vi "GT Get Kvff Filter.vi"(6 "pAccMax":dbl, 7 "pKvffFilterExp":i16, 8 "error in (no error)":errorcluster caption="错误输入（无错误）", 9 "index":i16, 10 "control":i16, 11 "cardNum":i16) -> (0 "error out":errorcluster caption="错误输出", 3 "function return":i16, 4 "pAccMax out":dbl, 5 "pKvffFilterExp out":i16)   [LabVIEW 2020, in "gts.lvlib"]
doc: "GT_API GT_GetKvffFilter(short cardNum,short control,short index,short *pKvffFilterExp,double *pAccMax);"
uses:
  gts.lvlib
  dll/32bit/multi_card/gts.dll
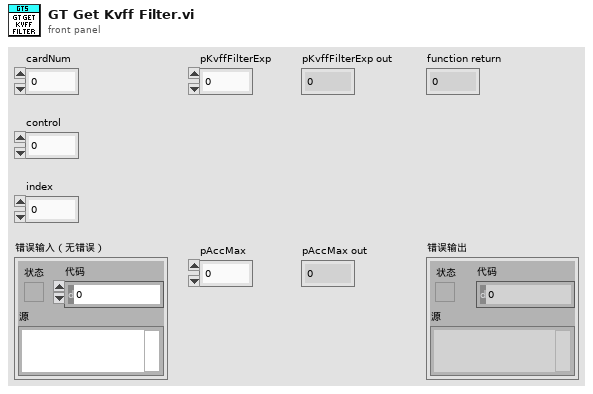
[diagram p1: front panel]
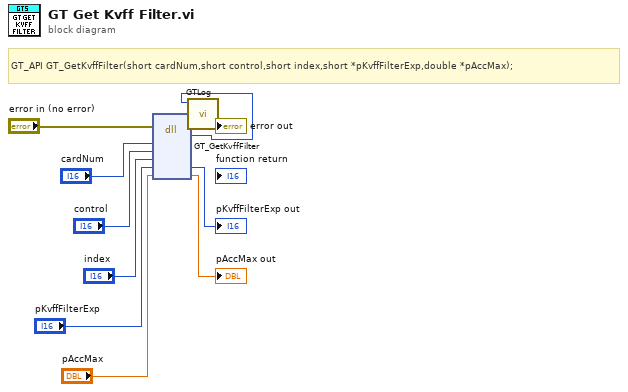
[diagram p0: block diagram]
diagram:
  # "GT_API GT_GetKvffFilter(short cardNum,short control,short index,short *pKvffFilterExp,double *pAccMax);"
  n1 = dll-call lib="C:/1228/dll/32bit/multi_card/gts.dll" fn="GT_GetKvffFilter"(error in="error in (no error)", "cardNum"="cardNum", "control"="control", "index"="index", "pKvffFilterExp"="pKvffFilterExp", "pAccMax"="pAccMax") -> (error out=w3:errorcluster, w1:i16, "pKvffFilterExp"=→"pKvffFilterExp out":i16, "pAccMax"=→"pAccMax out":dbl)  [unwired: 5 in, 1 out]
  n2 = call "GTLog.vi"("error in (no error)"=w3, "Numeric"=w1) -> ("error out"=→"error out":errorcluster)  [unwired: 9 in]
